vi "DSF.Engine.Buffer Converter.Set Channels Buffer.vi"(10 "channels buffer":dbl[](array[numeric]), 11 "Buffer Converter in":refnum<class "Buffer Converter.lvclass">) -> (3 "Buffer Converter out":refnum<class "Buffer Converter.lvclass">)   [LabVIEW 2017, in "DSF.Engine.lvlib" / "Buffer Converter.lvclass"]
uses:
  Buffer Converter.lvclass
  Buffer Converter.lvclass/Buffer Converter.ctl
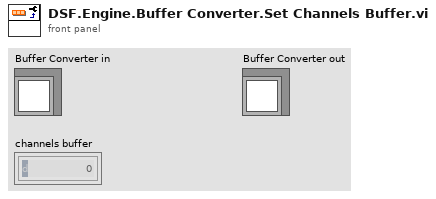
[diagram p1: front panel]
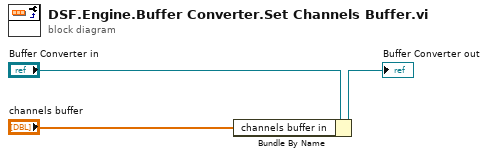
[diagram p0: block diagram]
diagram:
  n1 = Bundle By Name(cluster="Buffer Converter in", "channels buffer in"="channels buffer") -> (→"Buffer Converter out":refnum<class "Buffer Converter.lvclass">)
